vi "Add Project Item.vi"(8 "error in (no error)":errorcluster, 10 "Folder Location Ref":refnum<vi>, 11 "DMA Loop in":refnum<class "DMA Loop.lvclass">) -> (0 "error out":errorcluster, 3 "DMA Loop out":refnum<class "DMA Loop.lvclass">)   [LabVIEW 2015, in "DMA Loop.lvclass"]
uses:
  DMA Loop.lvclass
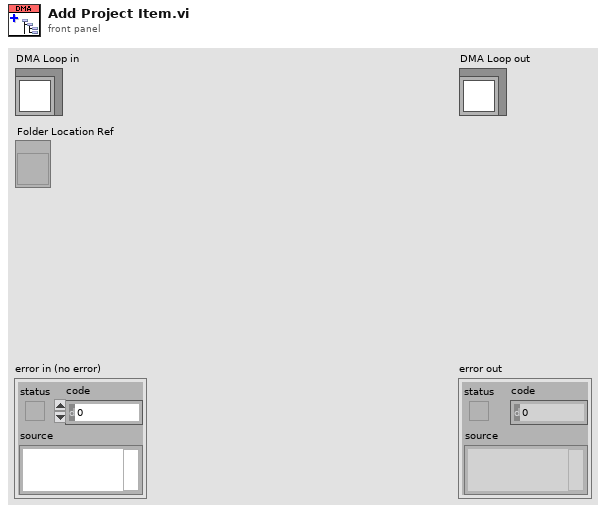
[diagram p1: front panel]
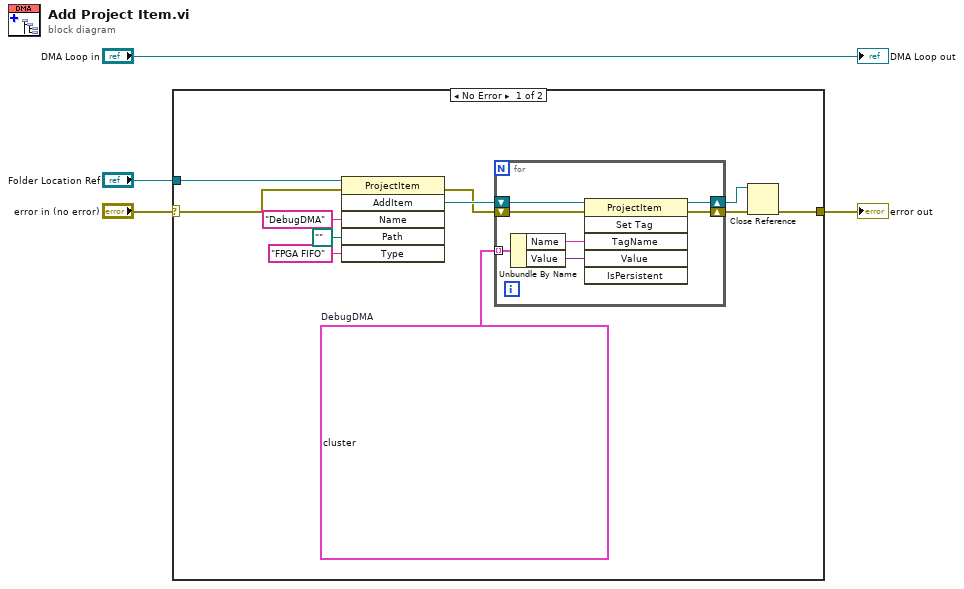
[diagram p0: block diagram]
diagram:
  n1 = case shown="No Error" "error in (no error)" {
    selector: "error in (no error)" -> [w7 w23]
    tunnel: [w6 w23] -> w3
    tunnel: "Folder Location Ref" -> [w5 _]
    frame No Error {
      w12 = cluster{"Name":string, "Value":variant}[] [{"Name"="Actual Number of Elements", "Value"=variant(u32 1023)}, {"Name"="Arbitration for Read", "Value"=variant(u32 1)}, {"Name"="Arbitration for Write", "Value"=variant(u32 1)}, {"Name"="Control Logic", "Value"=variant(u32 0)}, {"Name"="Data Type", "Value"=variant(u32 11)}, {"Name"="Disable on Overflow/Underflow", "Value"=variant(bool FALSE)}, {"Name"="fifo.configuration", "Value"=variant(string "\"ControlLogic=0;NumberOfElements=1023;Type=2;ReadArbs=Arbitrate if Multiple Requestors Only;ElementsPerRead=1;WriteArbs=Arbitrate if Multiple Requestors Only;ElementsPerWrite=1;Implementation=2;FIFO;DataType=100080000000000100094009000353474C000100000000000000000000;DisableOnOverflowUnderflow=FALSE\"")}, {"Name"="fifo.configured", "Value"=variant(bool TRUE)}, {"Name"="fifo.projectItemValid", "Value"=variant(bool TRUE)}, {"Name"="fifo.valid", "Value"=variant(bool TRUE)}, {"Name"="fifo.version", "Value"=variant(i32 12)}, {"Name"="FPGA.PersistentID", "Value"=variant(string "{43D2C6D9-9E30-4F2C-9E9A-27A6F06ED45E}")}, {"Name"="Local", "Value"=variant(bool FALSE)}, {"Name"="Memory Type", "Value"=variant(u32 2)}, {"Name"="Number Of Elements Per Read", "Value"=variant(u32 1)}, {"Name"="Number Of Elements Per Write", "Value"=variant(u32 1)}, {"Name"="Requested Number of Elements", "Value"=variant(u32 1023)}, {"Name"="Type", "Value"=variant(u32 2)}, {"Name"="Type Descriptor", "Value"=variant(string "100080000000000100094009000353474C000100000000000000000000")}]  # DebugDMA
      n2 = invoke class="ProjectItem" method="AddItem"(reference=w5, error in=w7, "Name"="DebugDMA", "Path"=path "", "Type"="FPGA FIFO") -> (error out=w10:errorcluster, "AddItem"=w13:refnum<vi>)  [unwired: 1 in, 4 out]
      n3 = for {
        shift-right: [w17] -> w8
        shift-left: w10 -> [w21]
        tunnel: w12 -> [w20] mode=indexing
        shift-right: [w16] -> w9
        shift-left: w13 -> [w22]
        n4 = Unbundle By Name(w20) -> ("Name"=w19:string, "Value"=w18:variant)
        n5 = invoke class="ProjectItem" method="Set Tag"(reference=w22, error in=w21, "TagName"=w19, "Value"=w18) -> (reference out=w16:refnum<vi>, error out=w17:errorcluster)  [unwired: 2 in, 4 out]
      }
      n6 = Close Reference(reference=w9, error in (no error)=w8) -> (error out=w6:errorcluster)
    }
    frame Error {
    }
  }
  "error out" <- w3
  "DMA Loop out" <- "DMA Loop in"
